vi "excersize 3.1.vi"() -> ()   [LabVIEW 2014]
panel:
  in  "current temp 2":dbl
  out "Warning Text":string
  out "Warning?":bool
  in  "Min Temp":dbl
  in  "Max temp":dbl
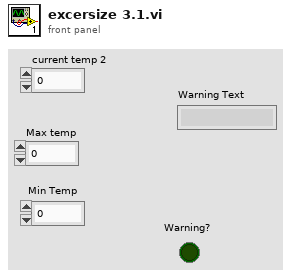
[diagram p1: front panel]
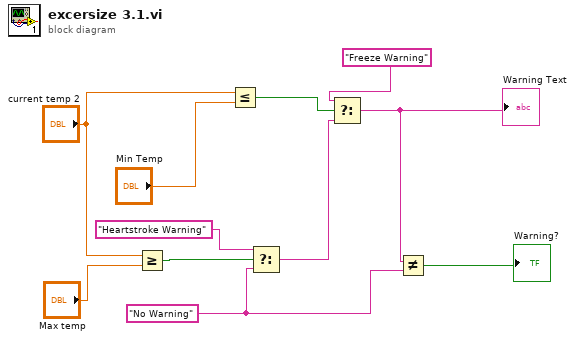
[diagram p0: block diagram]
diagram:
  w3 = "No Warning"
  n1 = Greater Or Equal?(x="current temp 2", y="Max temp") -> (x >= y?=w8:bool)
  n2 = Less Or Equal?(x="current temp 2", y="Min Temp") -> (x <= y?=w7:bool)
  n3 = Select(t="Heartstroke Warning", s=w8, f=w3) -> (s? t:f=w4:string)
  n4 = Select(t="Freeze Warning", s=w7, f=w4) -> (s? t:f=w2:string)
  "Warning Text" <- w2
  n5 = Not Equal?(x=w2, y=w3) -> (x != y?=→"Warning?":bool)
